vi "TDMSAdv getCurrentPath.vi"(8 "error in (no error)":errorcluster, 11 "TDMSAdv in":refnum<class "TDMSAdv.lvclass">) -> (0 "error out":errorcluster, 2 "currFIlePath":path, 3 "TDMSAdv out":refnum<class "TDMSAdv.lvclass">)   [LabVIEW 2018, in "TDMSAdv.lvclass"]
uses:
  TDMSAdv.lvclass
  TDMSAdv.lvclass/TDMSAdv.ctl
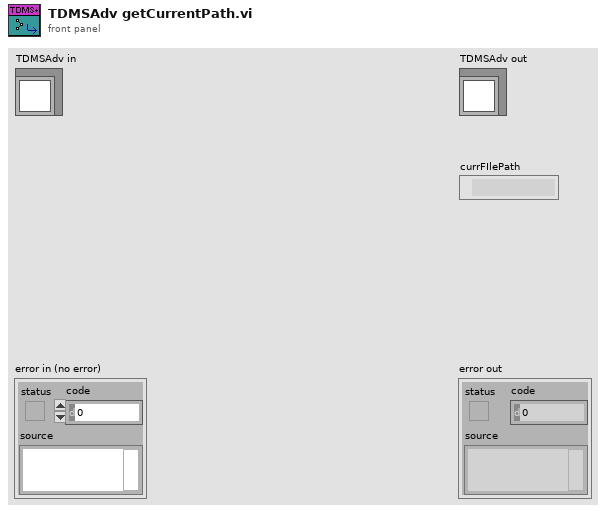
[diagram p1: front panel]
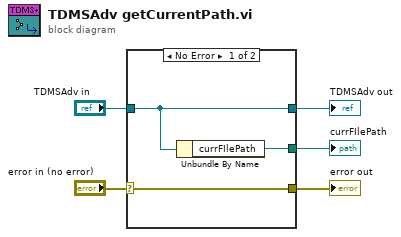
[diagram p0: block diagram]
diagram:
  n1 = case shown="No Error" "error in (no error)" {
    selector: "error in (no error)" -> [w8 w10]
    tunnel: [w8 w10] -> w4
    tunnel: [w7 w9] -> w2
    tunnel: "TDMSAdv in" -> [w7 w9]
    tunnel: [w6 _] -> w1
    frame No Error {
      n2 = Unbundle By Name(w7) -> ("currFIlePath"=w6:path)
    }
    frame Error {
    }
  }
  "error out" <- w4
  "TDMSAdv out" <- w2
  "currFIlePath" <- w1
